vi "Camera_Config_Specific_Attributes.vi"(4 "Crop?":bool, 5 "Camera":T1, 6 "Detect Movement":bool, 8 "error in (no error)":errorcluster, 10 "Refnum in":T2, 11 "input cluster":T3={"system"={"info"={"menuSelect"=0, "version"=0, "serial"="", "captureActive"=FALSE, "captureBegin"=FALSE, "emptyAndRefill"=FALSE}, "userInfo"={"operatorName"="", "date"=timestamp(2713993200 s since 1904-01-01)}, "camera"={"exposureTime"=0, "aperture"=enum."Item 0", "framerate"=0, "framerateMax"=0, "legacyAttributes"=FALSE}}, "connections"={"arduino"={"connection"="", "status"=FALSE, "openState"=FALSE, "emptyStart"=0}, "pump"={"connection"="", "status"=FALSE, "command"="", "dispenseSpeed"=0, "flushSize"=0}, "camera"={"cam1"={"connection"="", "status"=FALSE}, "cam2"={"connection"="", "status"=FALSE}}}, "queue"={"process"={"cam1"=refnum, "cam2"=refnum, "queueSize"=0}, "save"={"cam1"=refnum, "cam2"=refnum, "queueSize"=0}, "overloadThreshold"=0}, "imageProcess"={"cam1"={"preAllocation"={"image"=refnum, "originalDisplay"=refnum, "originalRgb"=refnum, "binary"=refnum, "save"=refnum, "calibrationFull"=refnum, "calibrationDetect"=refnum}, "calibration"={"pathFull"=path "", "pathDetect"=path "", "ROI"={"Left"=0, "Top"=0, "Right"=0, "Bottom"=0, "Rotation"=0.0}}}, "cam2"={"preAllocation"={"image"=refnum, "originalDisplay"=refnum, "originalRgb"=refnum, "binary"=refnum, "save"=refnum, "calibrationFull"=refnum, "calibrationDetect"=refnum}, "calibration"={"pathFull"=path "", "pathDetect"=path "", "ROI"={"Left"=0, "Top"=0, "Right"=0, "Bottom"=0, "Rotation"=0.0}}}, "process"={"planeExtract"=refnum, "planeSubtract"=refnum, "cropMask"=refnum}, "detection"={"sampleTimeout"=0, "sizeThreshold"=0, "detectionRegionPct"=0.0}}, "sampleData"={"sampleId"="", "projectId"="", "voucherID"="", "speciesName"="", "collectionDate"=timestamp(2713993200 s since 1904-01-01), "sampleStation"="", "location"="", "lat"=0.0, "lon"=0.0, "determiner"="", "sex"="", "otherNotes"=""}, "Session In"=""} {"sampleData"."collectionDate" format="%<%Y-%m-%d>T"; "imageProcess"."detection"."sizeThreshold" min=1; "imageProcess"."cam2"."calibration"."ROI"."Rotation" format="%.2f"; "imageProcess"."cam2"."calibration"."ROI"."Left" scale=0.0..1024.0; "imageProcess"."cam2"."calibration"."ROI"."Right" scale=0.0..1024.0; "imageProcess"."cam1"."calibration"."ROI"."Rotation" format="%.2f"; "imageProcess"."cam1"."calibration"."ROI"."Left" scale=0.0..1024.0; "imageProcess"."cam1"."calibration"."ROI"."Right" scale=0.0..1024.0; "queue"."overloadThreshold" min=1; "queue"."save"."queueSize" min=1; "queue"."process"."queueSize" min=1; "connections"."pump"."flushSize" min=1; "connections"."pump"."dispenseSpeed" min=1; "system"."camera"."framerateMax" min=1; "system"."userInfo"."date" format="%<%Y-%m-%dT%H:%M:%S+%z>T"; "system"."info"."version" items=["Standard", "XL"]; "system"."info"."menuSelect" items=["Session Data", "Extended Setup", "Buffer", "Camera", "Dispenser", "Stats", "Connections"]}) -> (0 "error out":errorcluster, 3 "Refnum out":T2)   [LabVIEW 2022 SP3]
uses:
  <vilib>/userdefined/High Color/IMAQdx.ctl
  controls/Data.ctl
  <vilib>/vision/Image Controls.llb/IMAQ Image.ctl
  Camera_ID.ctl
  <resource>/objmgr/imaqdx.rc
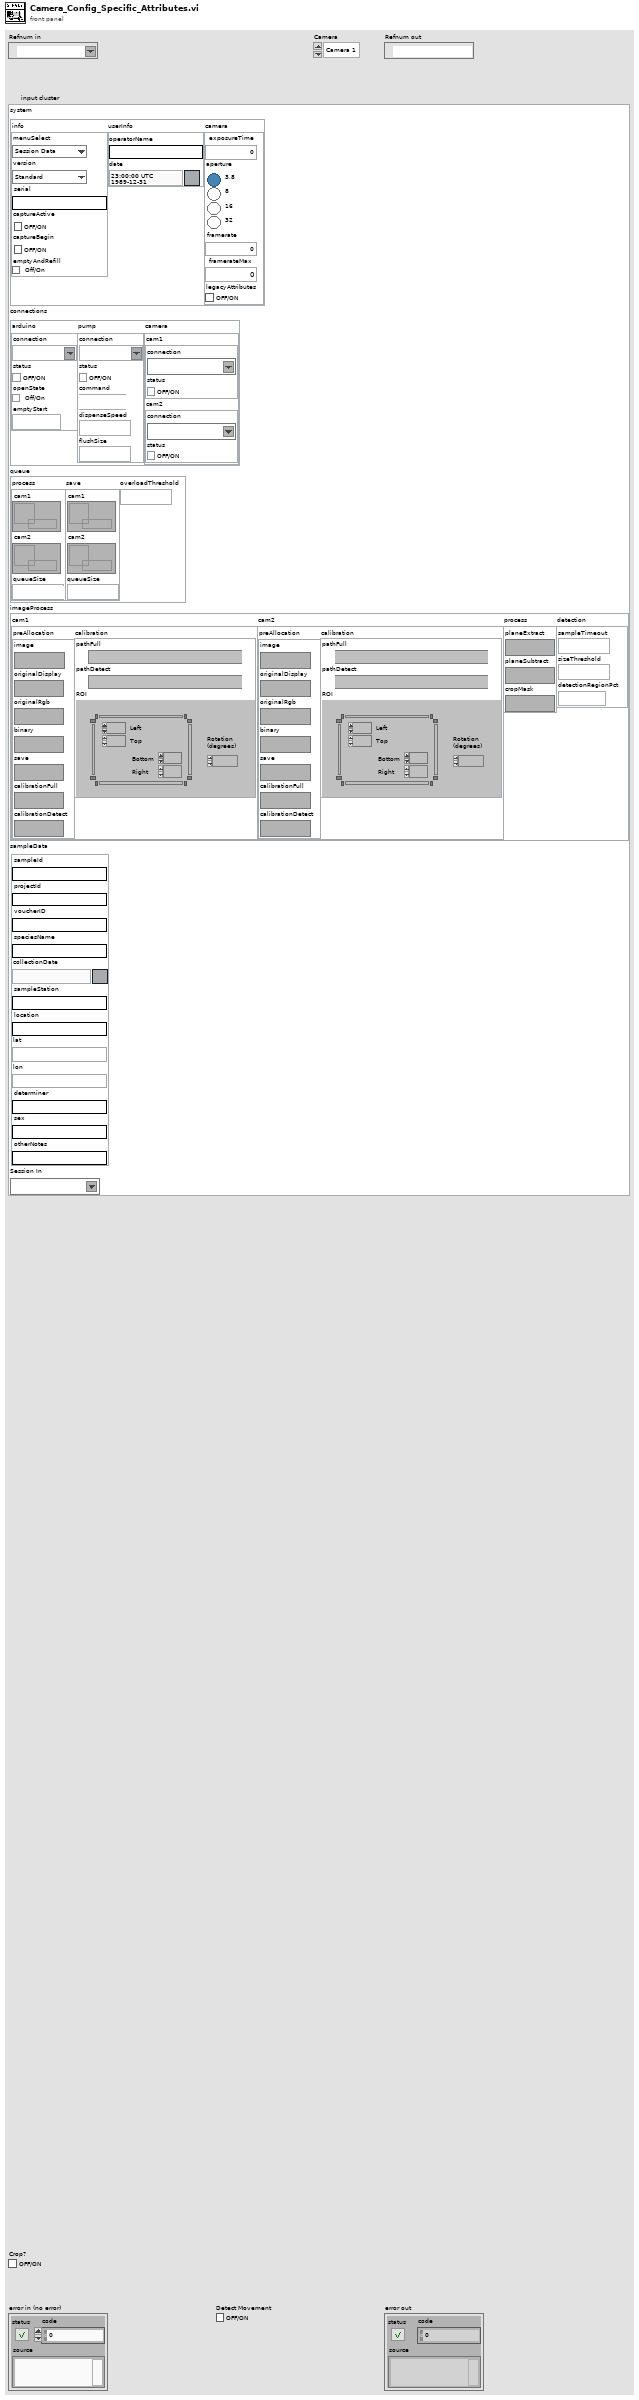
[diagram p1: front panel]
types:
  T1 = typedef "Camera_ID.ctl" = enum16{"Camera 1", "Camera 2"}
  T2 = typedef "IMAQdx.ctl" = refnum<k21>
  T3 = typedef "Data.ctl" = cluster{"system":cluster{"info":cluster{"menuSelect":u16, "version":u16, "serial":string, "captureActive":bool, "captureBegin":bool, "emptyAndRefill":bool}, "userInfo":cluster{"operatorName":string, "date":timestamp}, "camera":cluster{"exposureTime":i32, "aperture":enum32{"Item 0", "Item 1", "Item 2", "Item 3"}, "framerate":i32, "framerateMax":i32, "legacyAttributes":bool}}, "connections":cluster{"arduino":cluster{"connection":refnum<visa-resource-name>, "status":bool, "openState":bool, "emptyStart":u32}, "pump":cluster{"connection":refnum<visa-resource-name>, "status":bool, "command":string, "dispenseSpeed":i32, "flushSize":i32}, "camera":cluster{"cam1":cluster{"connection":T2, "status":bool}, "cam2":cluster{"connection":T2, "status":bool}}}, "queue":cluster{"process":cluster{"cam1":refnum<queue>, "cam2":refnum<queue>, "queueSize":i32}, "save":cluster{"cam1":refnum<queue>, "cam2":refnum<queue>, "queueSize":i32}, "overloadThreshold":i32}, "imageProcess":cluster{"cam1":cluster{"preAllocation":cluster{"image":T4, "originalDisplay":T4, "originalRgb":T4, "binary":T4, "save":T4, "calibrationFull":T4, "calibrationDetect":T4}, "calibration":cluster{"pathFull":path, "pathDetect":path, "ROI":T5}}, "cam2":cluster{"preAllocation":cluster{"image":T4, "originalDisplay":T4, "originalRgb":T4, "binary":T4, "save":T4, "calibrationFull":T4, "calibrationDetect":T4}, "calibration":cluster{"pathFull":path, "pathDetect":path, "ROI":T5}}, "process":cluster{"planeExtract":T4, "planeSubtract":T4, "cropMask":T4}, "detection":cluster{"sampleTimeout":i32, "sizeThreshold":i32, "detectionRegionPct":dbl}}, "sampleData":cluster{"sampleId":string, "projectId":string, "voucherID":string, "speciesName":string, "collectionDate":timestamp, "sampleStation":string, "location":string, "lat":dbl, "lon":dbl, "determiner":string, "sex":string, "otherNotes":string}, "Session In":T2}
  T4 = typedef "IMAQ Image.ctl" = refnum<image>
  T5 = typedef "IMAQ Rectangle" = cluster{"Left":i32, "Top":i32, "Right":i32, "Bottom":i32, "Rotation":dbl}
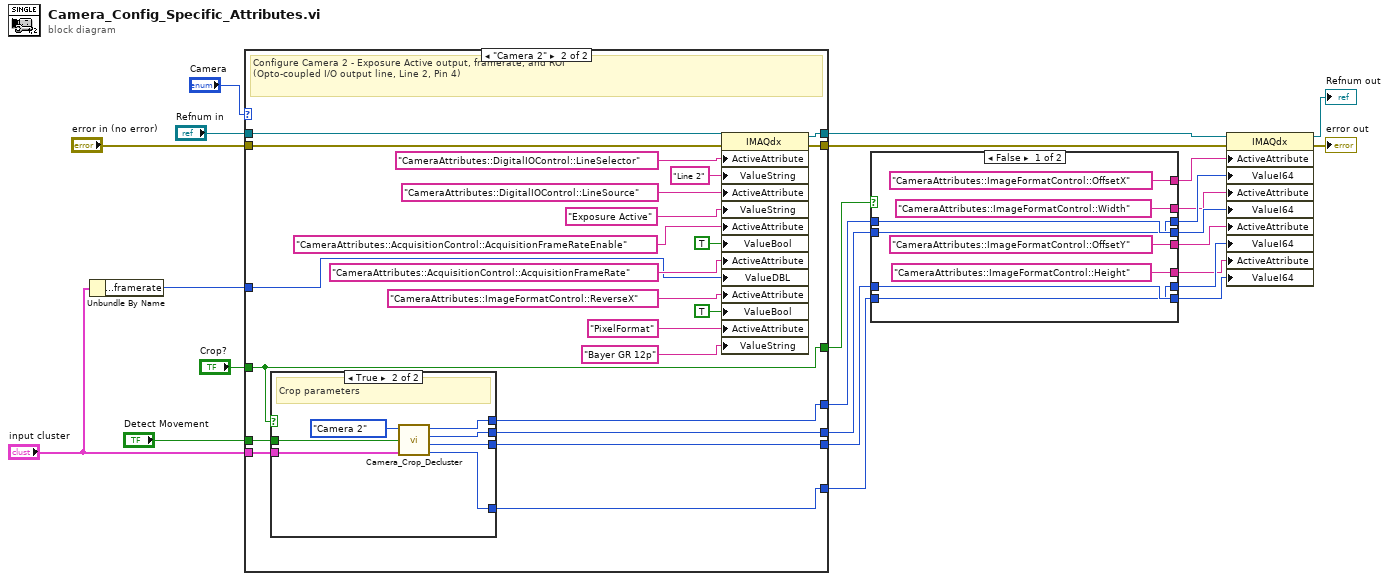
[diagram p0: block diagram]
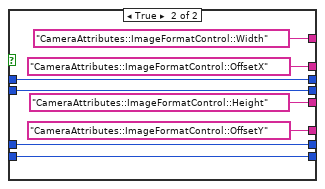
[diagram p2: hidden frame]
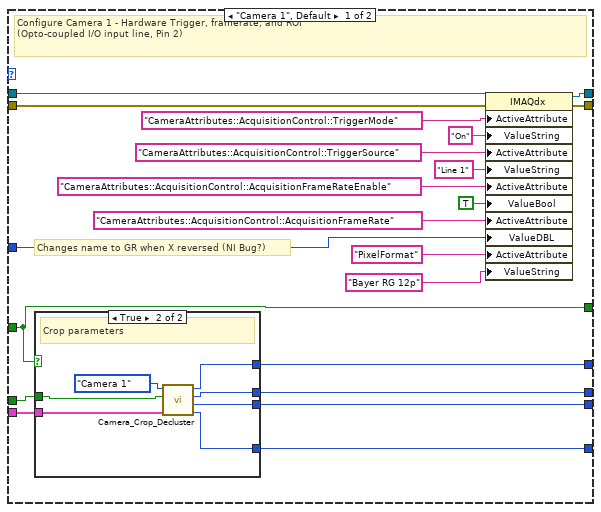
[diagram p3: hidden frame]
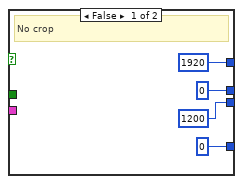
[diagram p4: hidden frame]
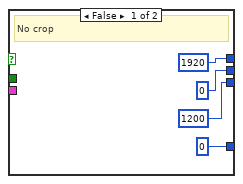
[diagram p5: hidden frame]
diagram:
  n1 = Unbundle By Name("input cluster") -> ("system.camera.framerate"=w1:i32)
  n2 = case shown="\"Camera 2\"" "Camera" {
    tunnel: "Refnum in" -> [w45 w66]
    tunnel: [w44 w65] -> w11
    tunnel: [w43 w64] -> w4
    tunnel: w1 -> [w35 w63]
    tunnel: [w33 w79] -> w17
    tunnel: [w34 w78] -> w14
    tunnel: [w31 w76] -> w19
    tunnel: [w32 w77] -> w15
    tunnel: "Crop?" -> [w30 w75]
    tunnel: [w30 w75] -> w12
    tunnel: "input cluster" -> [w29 w74]
    tunnel: "Detect Movement" -> [w28 w73]
    tunnel: "error in (no error)" -> [w27 w59]
    frame "Camera 1", Default {
      # "Changes name to GR when X reversed (NI Bug?)"
      # "Configure Camera 1 - Hardware Trigger, framerate, and ROI \n(Opto-coupled I/O input line, Pin 2)"
      n3 = case shown="True" w30 {
        tunnel: [i64 1920 w55] -> w34
        tunnel: [1200 w53] -> w33
        tunnel: [i64 0 w54] -> w32
        tunnel: [0 w52] -> w31
        tunnel: w29 -> [_ w51]
        tunnel: w28 -> [_ w50]
        frame False {
          # "No crop"
        }
        frame True {
          # "Crop parameters"
          n4 = call "Camera_Crop_Decluster.vi"("input cluster"=w51, "Detect Movement"=w50, "Camera"=Camera_ID."Camera 1") -> ("OffsetY"=w52:i64, "Height"=w53:i64, "OffsetX"=w54:i64, "Width"=w55:i64)  [unwired: 5 in]
        }
      }
      n5 = property class="IMAQdx"(reference=w45, error in=w27, "ActiveAttribute"="CameraAttributes::AcquisitionControl::TriggerMode", "ValueString"="On", "ActiveAttribute"="CameraAttributes::AcquisitionControl::TriggerSource", "ValueString"="Line 1", "ActiveAttribute"="CameraAttributes::AcquisitionControl::AcquisitionFrameRateEnable", "ValueBool"=TRUE, "ActiveAttribute"="CameraAttributes::AcquisitionControl::AcquisitionFrameRate", "ValueDBL"=w35, "ActiveAttribute"="PixelFormat", "ValueString"="Bayer RG 12p") -> (reference out=w44:T2, error out=w43:errorcluster)
    }
    frame "Camera 2" {
      # "Configure Camera 2 - Exposure Active output, framerate, and ROI\n(Opto-coupled I/O output line, Line 2, Pin 4)"
      n6 = case shown="True" w75 {
        tunnel: [i64 1200 w86] -> w79
        tunnel: [i64 1920 w88] -> w78
        tunnel: [i64 0 w87] -> w77
        tunnel: [i64 0 w85] -> w76
        tunnel: w74 -> [_ w90]
        tunnel: w73 -> [_ w84]
        frame False {
          # "No crop"
        }
        frame True {
          # "Crop parameters"
          n7 = call "Camera_Crop_Decluster.vi"("input cluster"=w90, "Detect Movement"=w84, "Camera"=Camera_ID."Camera 2") -> ("OffsetY"=w85:i64, "Height"=w86:i64, "OffsetX"=w87:i64, "Width"=w88:i64)  [unwired: 5 in]
        }
      }
      n8 = property class="IMAQdx"(reference=w66, error in=w59, "ActiveAttribute"="CameraAttributes::DigitalIOControl::LineSelector", "ValueString"="Line 2", "ActiveAttribute"="CameraAttributes::DigitalIOControl::LineSource", "ValueString"="Exposure Active", "ActiveAttribute"="CameraAttributes::AcquisitionControl::AcquisitionFrameRateEnable", "ValueBool"=TRUE, "ActiveAttribute"="CameraAttributes::AcquisitionControl::AcquisitionFrameRate", "ValueDBL"=w63, "ActiveAttribute"="CameraAttributes::ImageFormatControl::ReverseX", "ValueBool"=TRUE, "ActiveAttribute"="PixelFormat", "ValueString"="Bayer GR 12p") -> (reference out=w65:T2, error out=w64:errorcluster)
    }
  }
  n9 = case shown="False" w12 {
    tunnel: ["CameraAttributes::ImageFormatControl::Height" ("ActiveAttribute") "CameraAttributes::ImageFormatControl::OffsetY" ("ActiveAttribute")] -> w5
    tunnel: ["CameraAttributes::ImageFormatControl::OffsetY" ("ActiveAttribute") "CameraAttributes::ImageFormatControl::Height" ("ActiveAttribute")] -> w6
    tunnel: ["CameraAttributes::ImageFormatControl::Width" ("ActiveAttribute") "CameraAttributes::ImageFormatControl::OffsetX" ("ActiveAttribute")] -> w7
    tunnel: ["CameraAttributes::ImageFormatControl::OffsetX" ("ActiveAttribute") "CameraAttributes::ImageFormatControl::Width" ("ActiveAttribute")] -> w8
    tunnel: [w93 w102] -> w13
    tunnel: w14 -> [w94 w102]
    tunnel: w15 -> [w93 w101]
    tunnel: [w94 w101] -> w16
    tunnel: w17 -> [w92 w100]
    tunnel: [w91 w100] -> w18
    tunnel: w19 -> [w91 w99]
    tunnel: [w92 w99] -> w20
    frame False {
    }
    frame True {
    }
  }
  n10 = property class="IMAQdx"(reference=w11, error in=w4, "ActiveAttribute"=w8, "ValueI64"=w13, "ActiveAttribute"=w7, "ValueI64"=w16, "ActiveAttribute"=w6, "ValueI64"=w18, "ActiveAttribute"=w5, "ValueI64"=w20) -> (reference out=→"Refnum out":T2, error out=→"error out":errorcluster)
